vi "Day_File_Plotter.vi"() -> ()   [LabVIEW 2012]
uses:
  Anemometry/Anemometry Sub Vis/File/Setup_Filetype.ctl
panel:
  in  "Reload":bool
  out "Setup exists?":bool
  out "Plot 3 status":string
  out "Plot 2 status":string
  out "Plot 1 status":string
  out "Change Scale?":bool
  out "Min Memory":timestamp
  out "Max Memory":timestamp
  in  "Show Full Time?":bool
  in  "Max Time":timestamp format="%<%H:%M\n%x>T"
  in  "Min Time":timestamp format="%<%H:%M\n%x>T"
  out "Plot 3 Chs":string[](array[string])
  out "Plot 2 Chs":string[](array[string])
  out "Plot 1 Chs":string[](array[string])
  in  "Save plot number":T1(ring)
  in  "Data folder location":path
  in  "Save 3":bool
  in  "Save 2":bool
  in  "Save 1":bool
  in  "Averaging Time (min)":dbl=1.0 min=0.0 format="%#.2f"
  in  "End Date":timestamp format="%<%x>T"
  in  "Selector 1":i32[](listbox)
  in  "Search 1":string
  in  "Search 2":string
  in  "Search 3":string
  out "Last Updated":string
  out "Plot 3":cluster{"Times":dbl[], "Output array":dbl[]}[](graph)
  in  "Selector 3":i32[](listbox)
  out "Plot 2":cluster{"Times":dbl[], "Output array":dbl[]}[](graph)
  in  "Selector 2":i32[](listbox)
  in  "stop":bool
  out "Plot 1":cluster{dbl[], "Output array":dbl[]}[](graph)
  in  "History (days)":i32 min=0
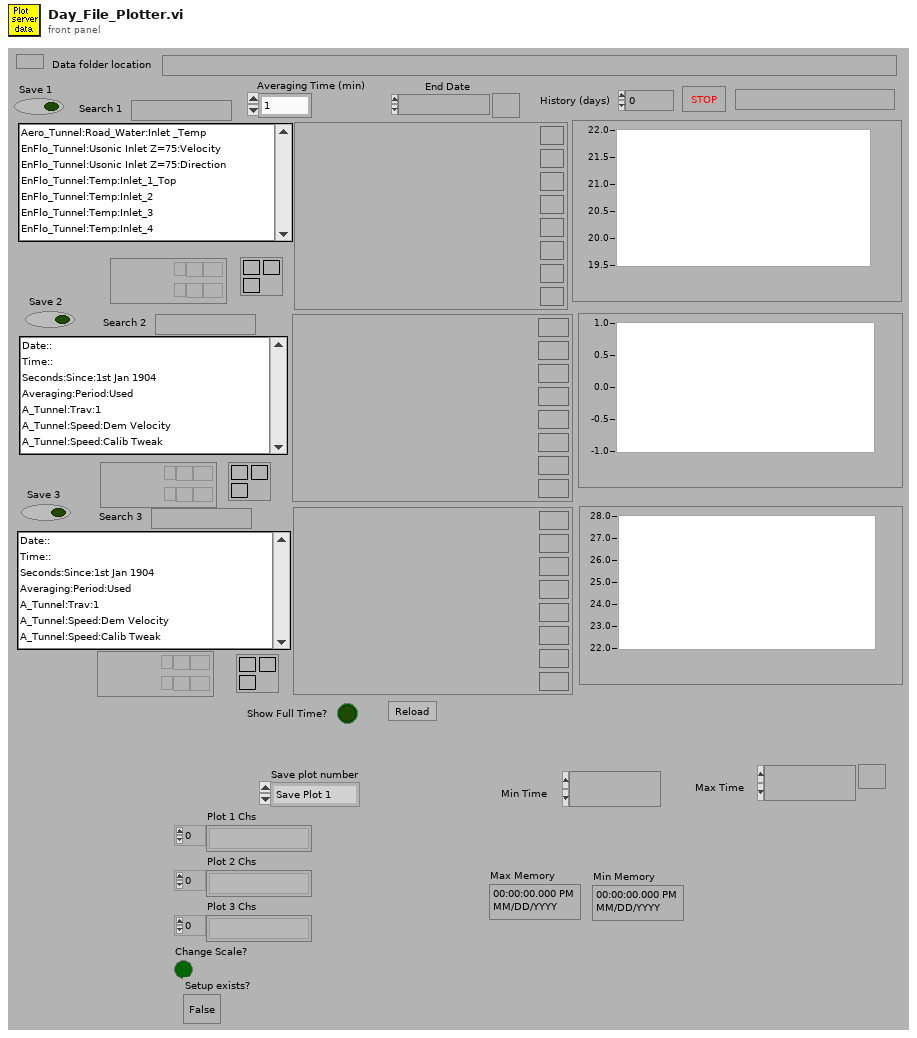
[diagram p1: front panel]
types:
  T1 = enum16{"Save Plot 1", "Save Plot 2", "Save Plot 3"}
  T2 = typedef "Setup_Filetype.ctl" = enum16{"Measurement Setups", "Calibration Setups", "General", "Results File Plotter Setups", "Speed Calib Tweaks"}
  T3 = enum32{"existing file", "new file", "new or existing file", "existing dir", "new dir", "new or existing dir", "existing file (use LLBs)", "new file (use LLBs)", "new or existing file (use LLBs)", "new or existing file or directory (use LLBs)"}
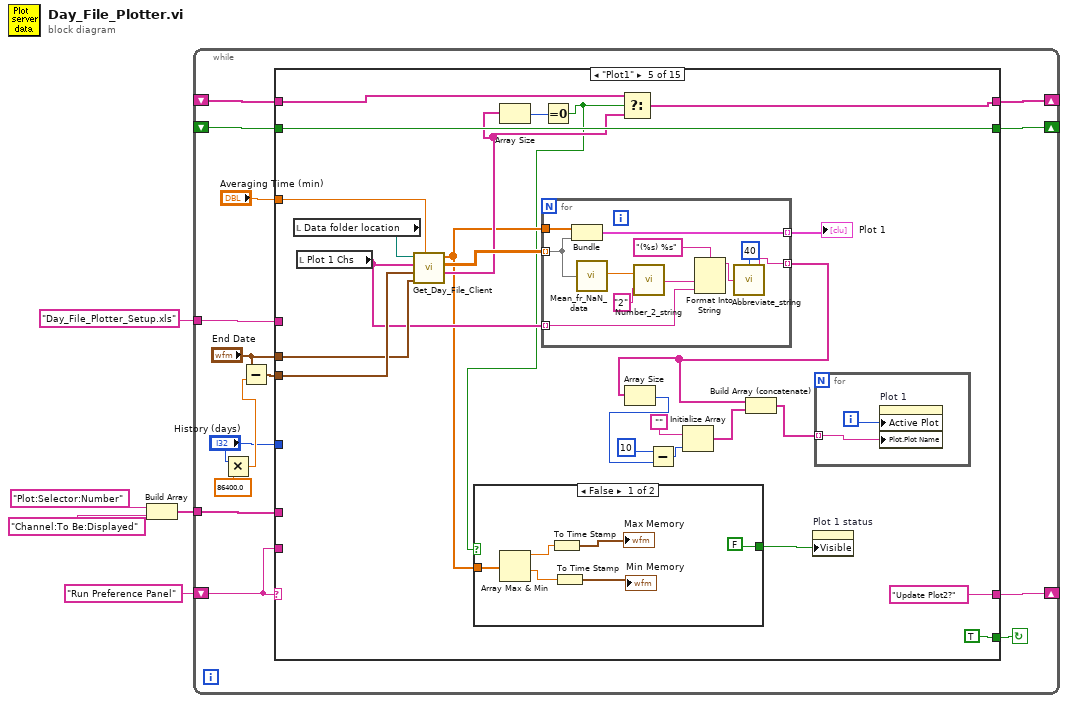
[diagram p0: block diagram]
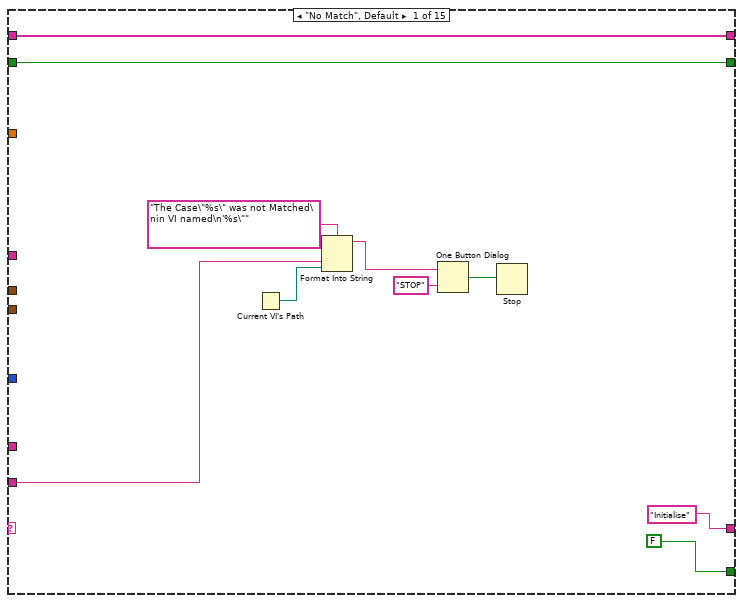
[diagram p2: hidden frame]
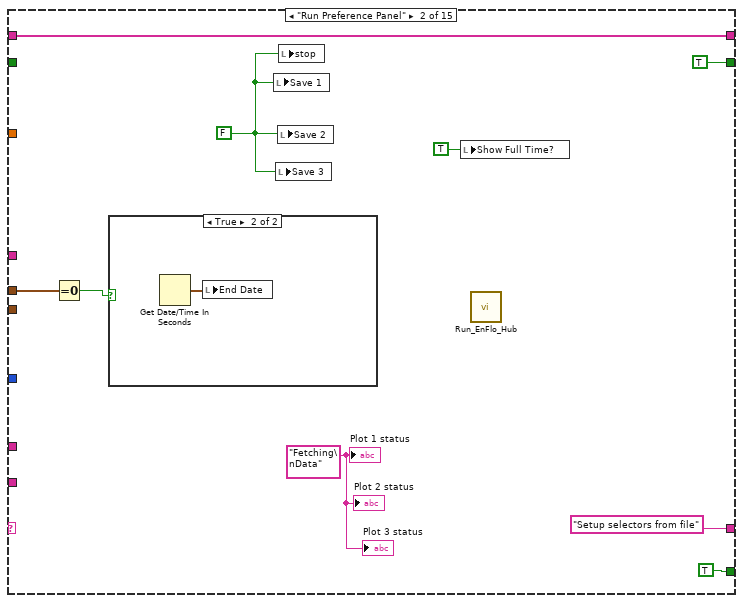
[diagram p3: hidden frame]
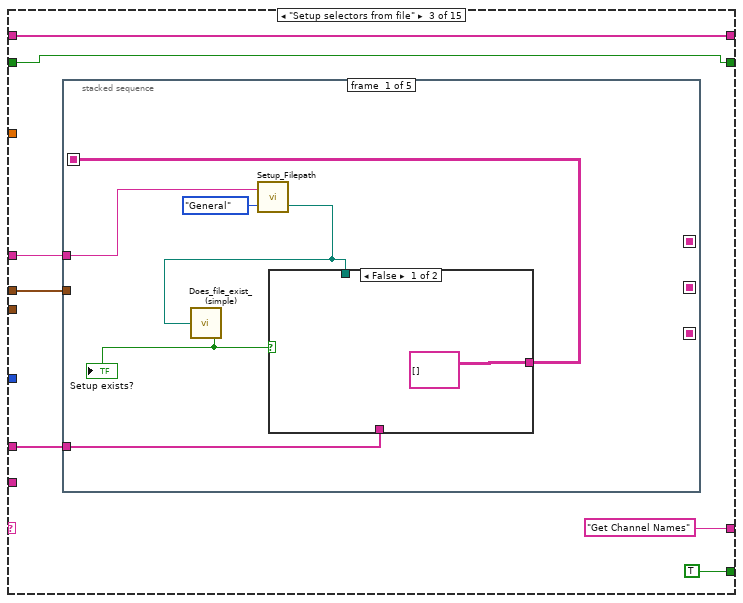
[diagram p5: hidden frame]
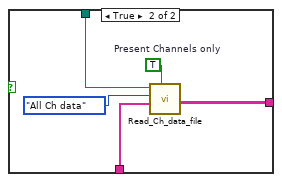
[diagram p6: hidden frame]
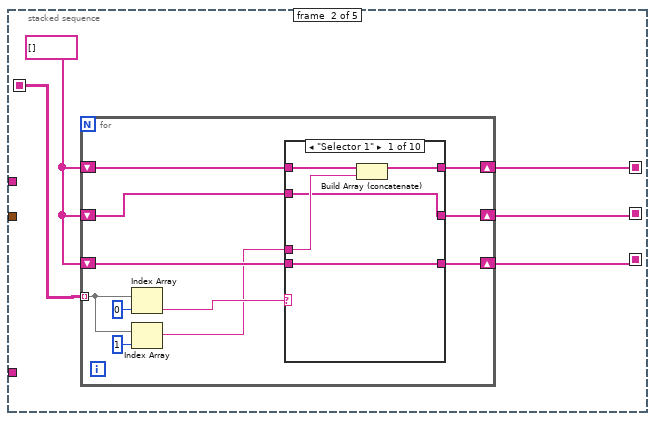
[diagram p7: hidden frame]
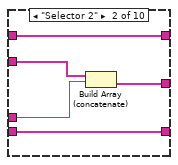
[diagram p8: hidden frame]
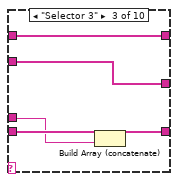
[diagram p9: hidden frame]
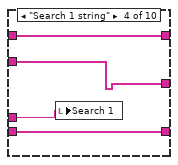
[diagram p10: hidden frame]
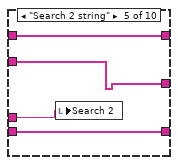
[diagram p11: hidden frame]
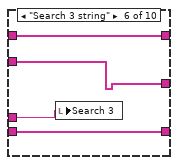
[diagram p12: hidden frame]
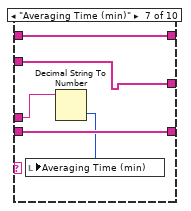
[diagram p13: hidden frame]
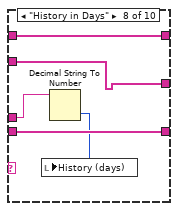
[diagram p14: hidden frame]
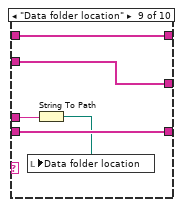
[diagram p15: hidden frame]
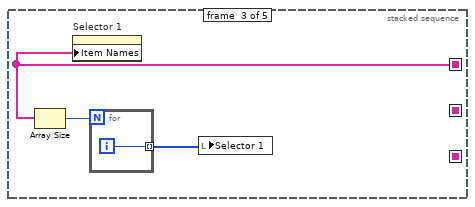
[diagram p17: hidden frame]
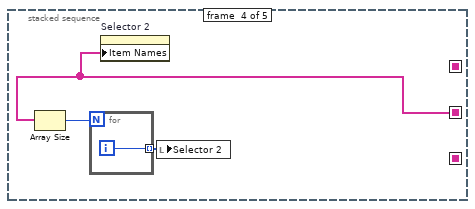
[diagram p18: hidden frame]
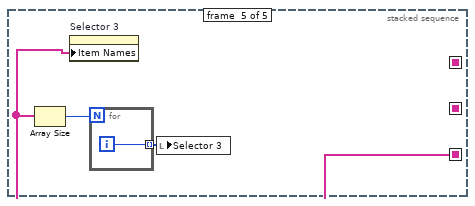
[diagram p19: hidden frame]
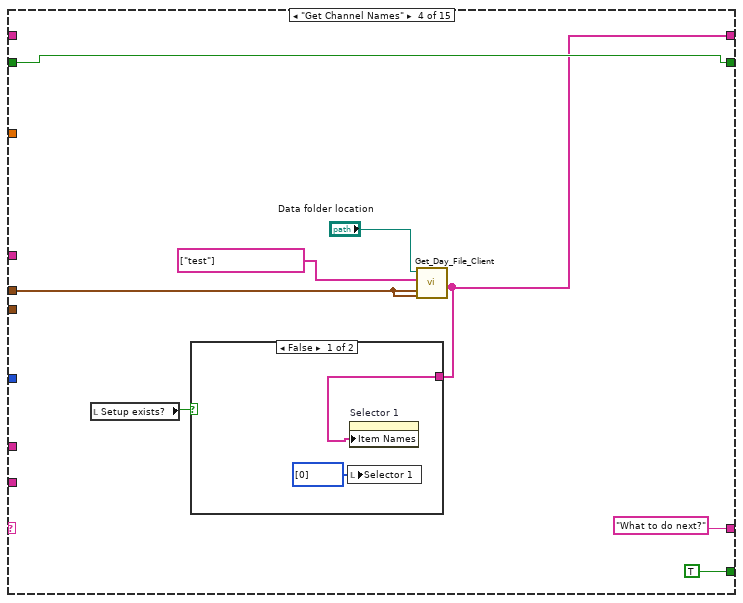
[diagram p20: hidden frame]
diagram:
  n1 = Build Array("Plot:Selector:Number", "Channel:To Be:Displayed") -> (w2:string[])
  n2 = while {
    shift-left: "Run Preference Panel" -> [w18]
    shift-right: [w19] -> _
    tunnel: w2 -> [w17]
    tunnel: "Day_File_Plotter_Setup.xls" -> [w16]
    shift-right: [w11] -> _
    shift-left: _ -> [w10]
    shift-right: [w7] -> _
    shift-left: _ -> [w6]
    stop <- w20 continue-if-true
    n3 = Multiply(x="History (days)", y=86400.0) -> (x*y=w14:dbl)
    n4 = Subtract(x="End Date", y=w14) -> (x-y=w13:timestamp)
    n5 = case shown="\"Plot1\"" w18 {
      tunnel: [FALSE TRUE TRUE TRUE TRUE TRUE TRUE TRUE TRUE TRUE TRUE TRUE TRUE TRUE w607] -> w20
      tunnel: ["Initialise" "Setup selectors from file" "Get Channel Names" "What to do next?" "Update Plot2?" "Update Plot3?" "Rescale plots?" "Update Plot1?" w314 w366 w420 w472 w568 w591 "Check for Zoom" ("t")] -> w19
      tunnel: w18 -> [w25 _ _ _ _ _ _ _ _ _ _ _ _ _ _]
      tunnel: w17 -> [_ _ w44 _ _ _ _ _ _ _ _ _ _ _ w614]
      tunnel: w16 -> [_ _ w45 _ _ _ _ _ _ _ _ _ _ _ w613]
      tunnel: w13 -> [_ _ _ _ w161 w206 w251 _ _ _ _ _ _ _ _]
      tunnel: "End Date" -> [_ w36 w42 w137 w160 w205 w250 _ _ _ _ _ w561 _ _]
      tunnel: [w22 TRUE w43 w138 w164 w209 w254 w282 w331 w384 w437 w473 w560 w590 w611] -> w11
      tunnel: w10 -> [w22 _ w43 w138 w164 w209 w254 w282 w331 w384 w437 w473 _ w589 w611]
      tunnel: "History (days)" -> [_ _ _ _ _ _ _ _ _ _ _ _ _ _ w605]
      tunnel: "Averaging Time (min)" -> [_ _ _ _ w163 w208 w253 _ _ _ _ _ w559 _ w610]
      tunnel: [w21 w34 w41 w134 w155 w200 w245 w283 w327 w380 w433 w474 w557 w596 w609] -> w7
      tunnel: w6 -> [w21 w34 w41 _ w157 w202 w247 w283 w327 w380 w433 w474 w557 w596 w609]
      frame "No Match", Default {
        n6 = Current VI's Path() -> (path=w24:path)
        n7 = Format Into String(format string="The Case\"%s\" was not Matched\nin VI named\n'%s\"" ("Format String"), w25, w24) -> (resulting string=w28:string)  [unwired: 2 in, 1 out]
        n8 = One Button Dialog(message=w28, button name ("OK")="STOP") -> (true=w26:bool)
        n9 = Stop(stop? (T)=w26) -> ()
      }
      frame "Run Preference Panel" {
        w31 = "Fetching\nData" ("Plot 1 status")
        w33 = FALSE
        n10 = Equal To 0?(x=w36) -> (x = 0?=w35:bool)
        n11 = case shown="True" w35 {
          frame False {
          }
          frame True {
            n12 = Get Date/Time In Seconds() -> (seconds since 1Jan1904=w40:timestamp)
            n13 = local write "End Date"(w40) -> ()
          }
        }
        n14 = local write "Save 1"(w33) -> ()
        n15 = local write "Save 3"(w33) -> ()
        n16 = local write "Save 2"(w33) -> ()
        n17 = local write "stop"(w33) -> ()
        n18 = local write "Show Full Time?"(TRUE ("Show Full Time?")) -> ()
        n19 = call "Run_EnFlo_Hub.vi"() -> ()  [unwired: 8 out]
        "Plot 1 status" <- w31
        "Plot 3 status" <- w31
        "Plot 2 status" <- w31
      }
      frame "Setup selectors from file" {
        n20 = stacked-sequence {
          seq-local: [w52 _ _ _ _] -> [_ w64 _ _ _]
          seq-local: [_ w62 _ _ _] -> [_ _ w123 _ _]
          seq-local: [_ w60 _ _ _] -> [_ _ _ w125 _]
          seq-local: [_ w61 _ _ _] -> [_ _ _ _ w129]
          tunnel: w45 -> [w49 _ _ _ _]
          tunnel: w44 -> [w53 _ _ _ _]
          tunnel: w42 -> [_ _ _ _ _]
          frame #0 {
            n21 = call "Setup_Filepath.vi"("Setup File Type"=Setup_Filetype."General", "Filename in"=w49) -> ("Filename Out"=w48:path)  [unwired: 1 out]
            n22 = call "Does_file_exist_(simple).vi"("Pathname"=w48) -> ("exists?"=w51:bool)
            "Setup exists?" <- w51
            n23 = case shown="False" w51 {
              tunnel: w48 -> [_ w59]
              tunnel: w53 -> [_ w58]
              tunnel: [string[][] [] ("Channel Values") w55] -> w52
              frame False {
              }
              frame True {
                w57 = TRUE  # Present Channels only
                n24 = call "Read_Ch_data_file.vi"("Present Channels only"=w57, "Present Channels"=w58, "Output"=enum16{"All Ch data", "The last few rows"}."All Ch data", "Filename"=w59) -> ("Channel Values"=w55:string[][])  [unwired: 1 in, 4 out]
              }
            }
          }
          frame #1 {
            w63 = string[] []
            n25 = for {
              shift-right: [w70] -> w62
              shift-left: w63 -> [w71]
              tunnel: w64 -> [w72] mode=indexing
              shift-right: [w68] -> w60
              shift-left: w63 -> [w69]
              shift-right: [w66] -> w61
              shift-left: w63 -> [w67]
              n26 = Index Array(array=w72, index=0 ("Index")) -> (element=w74:string)
              n27 = Index Array(array=w72, index=1 ("Index")) -> (element=w65:string)
              n28 = case shown="\"Selector 1\"" w74 {
                tunnel: w71 -> [w80 w85 w86 w94 w98 w102 w107 w108 w115 w120]
                tunnel: [w79 w85 w86 w94 w98 w102 w107 w108 w115 w120] -> w70
                tunnel: w65 -> [w78 w82 w88 w91 w95 w99 w104 w110 w114 _]
                tunnel: w69 -> [w77 w83 w87 w93 w97 w101 w106 w112 w117 w119]
                tunnel: [w77 w81 w87 w93 w97 w101 w106 w112 w117 w119] -> w68
                tunnel: w67 -> [w76 w84 w90 w92 w96 w100 w105 w111 w116 w118]
                tunnel: [w76 w84 w89 w92 w96 w100 w105 w111 w116 w118] -> w66
                frame "Selector 1" {
                  n29 = Build Array (concatenate)(w80, w78) -> (w79:string[])
                }
                frame "Selector 2" {
                  n30 = Build Array (concatenate)(w83, w82) -> (w81:string[])
                }
                frame "Selector 3" {
                  n31 = Build Array (concatenate)(w90, w88) -> (w89:string[])
                }
                frame "Search 1 string" {
                  n32 = local write "Search 1"(w91) -> ()
                }
                frame "Search 2 string" {
                  n33 = local write "Search 2"(w95) -> ()
                }
                frame "Search 3 string" {
                  n34 = local write "Search 3"(w99) -> ()
                }
                frame "Averaging Time (min)" {
                  n35 = Decimal String To Number(string=w104) -> (number=w103:i32)  [unwired: 3 out]
                  n36 = local write "Averaging Time (min)"(w103) -> ()
                }
                frame "History in Days" {
                  n37 = Decimal String To Number(string=w110) -> (number=w109:i32)  [unwired: 3 out]
                  n38 = local write "History (days)"(w109) -> ()
                }
                frame "Data folder location" {
                  n39 = String To Path(string=w114) -> (path=w113:path)
                  n40 = local write "Data folder location"(w113) -> ()
                }
                frame "No match", Default {
                }
              }
            }
          }
          frame #2 {
            n41 = Array Size(array=w123) -> (size(s)=w122:i32)
            n42 = property on="Selector 1" class="LstBox (strict)"("Item Names"=w123) -> ()  [unwired: 2 in, 2 out]
            n43 = for {
              N: w122 -> [_]
              tunnel: [w124] -> w121 mode=indexing
              i -> [w124]
            }
            n44 = local write "Selector 1"(w121) -> ()
          }
          frame #3 {
            n45 = Array Size(array=w125) -> (size(s)=w127:i32)
            n46 = for {
              N: w127 -> [_]
              tunnel: [w128] -> w126 mode=indexing
              i -> [w128]
            }
            n47 = property on="Selector 2" class="LstBox (strict)"("Item Names"=w125) -> ()  [unwired: 2 in, 2 out]
            n48 = local write "Selector 2"(w126) -> ()
          }
          frame #4 {
            n49 = Array Size(array=w129) -> (size(s)=w131:i32)
            n50 = property on="Selector 3" class="LstBox (strict)"("Item Names"=w129) -> ()  [unwired: 2 in, 2 out]
            n51 = for {
              N: w131 -> [_]
              tunnel: [w132] -> w130 mode=indexing
              i -> [w132]
            }
            n52 = local write "Selector 3"(w130) -> ()
          }
        }
      }
      frame "Get Channel Names" {
        n53 = local read "Setup exists?"() -> (w133:bool)
        n54 = call "Get_Day_File_Client.vi"("End time"=w137, "Start time"=w137, "Channel Names"=string[] ["test"], "Data folder location"="Data folder location") -> ("All Channel Names"=w134:string[])  [unwired: 1 in, 3 out]
        n55 = case shown="False" w133 {
          tunnel: w134 -> [w142 _]
          frame False {
            n56 = local write "Selector 1"(i32[] [0] ("Selector 1")) -> ()
            n57 = property on="Selector 1" class="LstBox (strict)"("Item Names"=w142) -> ()  [unwired: 2 in, 2 out]
          }
          frame True {
          }
        }
      }
      frame "Plot1" {
        n58 = local read "Data folder location"() -> (w162:path)
        n59 = local read "Plot 1 Chs"() -> (w147:string[])
        n60 = call "Get_Day_File_Client.vi"("Averaging Time (min)"=w163, "End time"=w160, "Start time"=w161, "Channel Names"=w147, "Data folder location"=w162) -> ("All Channel Names"=w156:string[], "Data"=w159:dbl[][], "Times"=w145:dbl[])  [unwired: 1 out]
        n61 = Array Size(array=w156) -> (size(s)=w158:i32)
        n62 = for {
          tunnel: w159 -> [w175] mode=indexing
          tunnel: [w184] -> w154 mode=indexing
          tunnel: w145 -> [w183]
          tunnel: [w179] -> w146 mode=indexing
          tunnel: w147 -> [w176] mode=indexing
          n63 = Bundle("Times"=w183, "Data"=w175) -> (w184:cluster{"Times":dbl[], "Data":dbl[]})  [unwired: 1 out]
          n64 = call "Mean_fr_NaN_data.vi"("Data"=w175) -> ("Mean value"=w174:dbl)  [unwired: 1 out]
          n65 = call "Number_2_string.vi"("precision"="2", "number"=w174) -> ("String"=w177:string)
          n66 = Format Into String(format string="(%s) %s", w177, w176) -> (resulting string=w180:string)  [unwired: 2 in, 1 out]
          n67 = call "Abbreviate_string.vi"("Input String"=w180, "Max String Length"=40) -> ("Output String"=w179:string)
        }
        "Plot 1" <- w154
        n68 = Equal To 0?(x=w158) -> (x = 0?=w144:bool)
        n69 = case shown="False" w144 {
          tunnel: w145 -> [w172 _]
          tunnel: [FALSE ("Visible") FALSE ("Visible")] -> w143
          frame False {
            n70 = Array Max & Min(array=w172) -> (max value=w171:dbl, min value=w169:dbl)  [unwired: 2 out]
            n71 = To Time Stamp(1:w171) -> (0:→"Max Memory":timestamp)
            n72 = To Time Stamp(1:w169) -> (0:→"Min Memory":timestamp)
          }
          frame True {
          }
        }
        n73 = Select(t=w157, s=w144, f=w156) -> (s? t:f=w155:string[])
        n74 = Array Size(array=w146) -> (size(s)=w152:i32)
        n75 = Subtract(x=10 ("dimension size"), y=w152) -> (x-y=w153:i32)
        n76 = Initialize Array("", w153) -> (w150:string[])
        n77 = Build Array (concatenate)(w146, w150) -> (w148:string[])
        n78 = property on="Plot 1 status" class="Str"("Visible"=w143) -> ()  [unwired: 2 in, 2 out]
        n79 = for {
          tunnel: w148 -> [w185] mode=indexing
          i -> [w186]
          n80 = property on="Plot 1" class="XYGraph (strict)"("Active Plot"=w186, "Plot.Plot Name"=w185) -> ()  [unwired: 2 in, 2 out]
        }
      }
      frame "Plot2" {
        n81 = local read "Plot 2 Chs"() -> (w193:string[])
        n82 = local read "Data folder location"() -> (w207:path)
        n83 = call "Get_Day_File_Client.vi"("Averaging Time (min)"=w208, "End time"=w205, "Start time"=w206, "Channel Names"=w193, "Data folder location"=w207) -> ("All Channel Names"=w201:string[], "Data"=w204:dbl[][], "Times"=w190:dbl[])  [unwired: 1 out]
        n84 = Array Size(array=w201) -> (size(s)=w203:i32)
        n85 = for {
          tunnel: w204 -> [w220] mode=indexing
          tunnel: [w229] -> w192 mode=indexing
          tunnel: w190 -> [w228]
          tunnel: [w224] -> w191 mode=indexing
          tunnel: w193 -> [w221] mode=indexing
          n86 = Bundle("Times"=w228, "Data"=w220) -> (w229:cluster{"Times":dbl[], "Data":dbl[]})  [unwired: 1 out]
          n87 = call "Mean_fr_NaN_data.vi"("Data"=w220) -> ("Mean value"=w219:dbl)  [unwired: 1 out]
          n88 = call "Number_2_string.vi"("precision"="2", "number"=w219) -> ("String"=w222:string)
          n89 = Format Into String(format string="(%s) %s", w222, w221) -> (resulting string=w225:string)  [unwired: 2 in, 1 out]
          n90 = call "Abbreviate_string.vi"("Input String"=w225, "Max String Length"=40) -> ("Output String"=w224:string)
        }
        "Plot 2" <- w192
        n91 = Equal To 0?(x=w203) -> (x = 0?=w189:bool)
        n92 = case shown="True" w189 {
          tunnel: w190 -> [w213 _]
          tunnel: [w212 w218] -> w188
          tunnel: FALSE -> [w212 w218]
          frame False {
            n93 = Array Max & Min(array=w213) -> (max value=w217:dbl, min value=w216:dbl)  [unwired: 2 out]
            n94 = To Time Stamp(1:w217) -> (0:w214:timestamp)
            n95 = To Time Stamp(1:w216) -> (0:w215:timestamp)
            n96 = local write "Max Memory"(w214) -> ()
            n97 = local write "Min Memory"(w215) -> ()
          }
          frame True {
          }
        }
        n98 = Array Size(array=w191) -> (size(s)=w198:i32)
        n99 = Select(t=w202, s=w189, f=w201) -> (s? t:f=w200:string[])
        n100 = Subtract(x=10 ("dimension size"), y=w198) -> (x-y=w199:i32)
        n101 = Initialize Array("", w199) -> (w196:string[])
        n102 = Build Array (concatenate)(w191, w196) -> (w194:string[])
        n103 = property on="Plot 2 status" class="Str"("Visible"=w188) -> ()  [unwired: 2 in, 2 out]
        n104 = for {
          tunnel: w194 -> [w230] mode=indexing
          i -> [w231]
          n105 = property on="Plot 2" class="XYGraph (strict)"("Active Plot"=w231, "Plot.Plot Name"=w230) -> ()  [unwired: 2 in, 2 out]
        }
      }
      frame "Plot3" {
        n106 = local read "Plot 3 Chs"() -> (w238:string[])
        n107 = local read "Data folder location"() -> (w252:path)
        n108 = call "Get_Day_File_Client.vi"("Averaging Time (min)"=w253, "End time"=w250, "Start time"=w251, "Channel Names"=w238, "Data folder location"=w252) -> ("All Channel Names"=w246:string[], "Data"=w249:dbl[][], "Times"=w235:dbl[])  [unwired: 1 out]
        n109 = Array Size(array=w246) -> (size(s)=w248:i32)
        n110 = for {
          tunnel: w249 -> [w265] mode=indexing
          tunnel: [w274] -> w237 mode=indexing
          tunnel: w235 -> [w273]
          tunnel: [w269] -> w236 mode=indexing
          tunnel: w238 -> [w266] mode=indexing
          n111 = Bundle("Times"=w273, "Data"=w265) -> (w274:cluster{"Times":dbl[], "Data":dbl[]})  [unwired: 1 out]
          n112 = call "Mean_fr_NaN_data.vi"("Data"=w265) -> ("Mean value"=w264:dbl)  [unwired: 1 out]
          n113 = call "Number_2_string.vi"("precision"="2", "number"=w264) -> ("String"=w267:string)
          n114 = Format Into String(format string="(%s) %s", w267, w266) -> (resulting string=w270:string)  [unwired: 2 in, 1 out]
          n115 = call "Abbreviate_string.vi"("Input String"=w270, "Max String Length"=40) -> ("Output String"=w269:string)
        }
        "Plot 3" <- w237
        n116 = Equal To 0?(x=w248) -> (x = 0?=w234:bool)
        n117 = case shown="True" w234 {
          tunnel: w235 -> [w258 _]
          tunnel: [w257 w263] -> w233
          tunnel: FALSE -> [w257 w263]
          frame False {
            n118 = Array Max & Min(array=w258) -> (max value=w262:dbl, min value=w261:dbl)  [unwired: 2 out]
            n119 = To Time Stamp(1:w262) -> (0:w259:timestamp)
            n120 = To Time Stamp(1:w261) -> (0:w260:timestamp)
            n121 = local write "Max Memory"(w259) -> ()
            n122 = local write "Min Memory"(w260) -> ()
          }
          frame True {
          }
        }
        n123 = Array Size(array=w236) -> (size(s)=w243:i32)
        n124 = Select(t=w247, s=w234, f=w246) -> (s? t:f=w245:string[])
        n125 = Subtract(x=10 ("dimension size"), y=w243) -> (x-y=w244:i32)
        n126 = Initialize Array("", w244) -> (w241:string[])
        n127 = Build Array (concatenate)(w236, w241) -> (w239:string[])
        n128 = property on="Plot 3 status" class="Str"("Visible"=w233) -> ()  [unwired: 2 in, 2 out]
        n129 = for {
          tunnel: w239 -> [w275] mode=indexing
          i -> [w276]
          n130 = property on="Plot 3" class="XYGraph (strict)"("Active Plot"=w276, "Plot.Plot Name"=w275) -> ()  [unwired: 2 in, 2 out]
        }
      }
      frame "Check for Zoom" {
        n131 = local read "Change Scale?"() -> (w278:bool)
        n132 = Or(x=w278, y="Show Full Time?") -> (x .or. y?=w277:bool)
        n133 = case shown="False" w277 {
          frame False {
            n134 = local read "Max Time"() -> (w290:timestamp)
            n135 = local read "Min Time"() -> (w291:timestamp)
            n136 = To Double Precision Float(number=w290) -> (double precision float=w289:dbl)
            n137 = To Double Precision Float(number=w291) -> (double precision float=w288:dbl)
            n138 = while {
              tunnel: w289 -> [w300]
              tunnel: w288 -> [w299]
              tunnel: [w293] -> w287
              tunnel: [w292] -> w286
              i -> [w302]
              stop <- w294 continue-if-true
              n139 = Increment(x=w302) -> (x+1=w301:i32)
              n140 = case shown="3" w301 {
                tunnel: [w305 w307 w310] -> w293
                tunnel: [w304 w306 w309] -> w292
                tunnel: [TRUE TRUE FALSE] -> w295
                frame 1, Default {
                  n141 = property on="Plot 1" class="XYGraph (strict)"() -> ("X Scale.Range:Maximum"=w305:dbl, "X Scale.Range:Minimum"=w304:dbl)  [unwired: 2 in, 2 out]
                }
                frame 2 {
                  n142 = property on="Plot 2" class="XYGraph (strict)"() -> ("X Scale.Range:Maximum"=w307:dbl, "X Scale.Range:Minimum"=w306:dbl)  [unwired: 2 in, 2 out]
                }
                frame 3 {
                  n143 = property on="Plot 3" class="XYGraph (strict)"() -> ("X Scale.Range:Maximum"=w310:dbl, "X Scale.Range:Minimum"=w309:dbl)  [unwired: 2 in, 2 out]
                }
              }
              n144 = Equal?(x=w300, y=w293) -> (x = y?=w297:bool)
              n145 = Equal?(x=w292, y=w299) -> (x = y?=w298:bool)
              n146 = And(x=w297, y=w298) -> (x .and. y?=w296:bool)
              n147 = And(x=w296, y=w295) -> (x .and. y?=w294:bool)
            }
            n148 = To Time Stamp(1:w287) -> (0:w284:timestamp)
            n149 = To Time Stamp(1:w286) -> (0:w285:timestamp)
            n150 = local write "Max Time"(w284) -> ()
            n151 = local write "Min Time"(w285) -> ()
          }
          frame True {
          }
        }
      }
      frame "Update Plot1?" {
        n152 = property on="Selector 1" class="LstBox (strict)"() -> ("Item Names"=w325:string[])  [unwired: 2 in, 2 out]
        n153 = case shown="True" "Save 1" {
          tunnel: ["Update Plot2?" "Save Plot" ("t")] -> w312
          frame False {
          }
          frame True {
            n154 = local write "Save plot number"(T1."Save Plot 1" ("Save plot number")) -> ()
          }
        }
        n155 = for {
          tunnel: w327 -> [w354]
          shift-right: [w349] -> w326
          shift-left: string[] [] -> [w350]
          tunnel: w325 -> [w352]
          tunnel: "Selector 1" -> [w351] mode=indexing
          n156 = Index Array(array=w352, index=w351) -> (element=w348:string)
          n157 = Search 1D Array(1D array=w354, element=w348) -> (index of element=w353:i32)  [unwired: 1 out]
          n158 = case shown="0, Default" w353 {
            tunnel: w353 -> [_ _]
            tunnel: w350 -> [w357 w358]
            tunnel: [w356 w358] -> w349
            tunnel: w348 -> [w355 _]
            frame 0, Default {
              n159 = Build Array (concatenate)(w357, w355) -> (w356:string[])
            }
            frame -1 {
            }
          }
        }
        "Plot 1 Chs" <- w326
        n160 = while {
          shift-right: [w359] -> w334
          shift-left: _ -> [w364]
          tunnel: [w364] -> w333
          shift-right: [w361] -> _
          shift-left: _ -> [w362]
          tunnel: w331 -> [w361]
          tunnel: [w360] -> w330
          tunnel: w326 -> [w359]
          stop <- FALSE continue-if-true
          n161 = Not Equal?(x=w362, y=w361) -> (x != y?=w360:bool)
        }
        n162 = Not Equal?(x=w333, y=w334) -> (x != y?=w332:bool)
        n163 = And(x=w331, y=w330) -> (x .and. y?=w329:bool)
        n164 = Compound Arithmetic op=OR(w329, w332) -> (w313:bool)
        n165 = case shown="True" w313 {
          tunnel: [w336 "Plot1"] -> w314
          tunnel: w312 -> [w336 _]
          frame False {
          }
          frame True {
            n166 = property on="Plot 1 status" class="Str"("Visible"=TRUE) -> ()  [unwired: 2 in, 2 out]
          }
        }
        n167 = call "Selection_with_Search.vi"("Selected Channel Names"=w326, "Search String"="Search 1", "All Channel Names"=w327) -> ("Item Names"=w322:string[])
        n168 = for {
          tunnel: w322 -> [w347]
          tunnel: w326 -> [w346] mode=indexing
          tunnel: [w345] -> w323 mode=indexing
          n169 = Search 1D Array(1D array=w347, element=w346) -> (index of element=w345:i32)  [unwired: 1 out]
        }
        n170 = Not Equal?(x=w322, y=w325) -> (x != y?=w324:bool)
        n171 = To Double Precision Float(number="Max Time") -> (double precision float=w317:dbl)
        n172 = To Double Precision Float(number="Min Time") -> (double precision float=w315:dbl)
        n173 = case shown="True" w324 {
          tunnel: w323 -> [_ w344]
          tunnel: w322 -> [_ w343]
          frame False {
          }
          frame True {
            n174 = local write "Selector 1"(w344) -> ()
            n175 = property on="Selector 1" class="LstBox (strict)"("Item Names"=w343, "Top Row"=0) -> ()  [unwired: 2 in, 2 out]
          }
        }
        n176 = property on="Plot 1" class="XYGraph (strict)"("X Scale.Range:Maximum"=w317, "X Scale.Range:Minimum"=w315) -> ()  [unwired: 2 in, 2 out]
      }
      frame "Update Plot2?" {
        n177 = property on="Selector 2" class="LstBox (strict)"() -> ("Item Names"=w375:string[])  [unwired: 2 in, 2 out]
        n178 = case shown="True" "Save 2" {
          tunnel: ["Update Plot3?" "Save Plot" ("t")] -> w365
          frame False {
          }
          frame True {
            n179 = local write "Save plot number"(T1."Save Plot 2" ("Save plot number")) -> ()
          }
        }
        n180 = for {
          tunnel: w380 -> [w407]
          shift-right: [w402] -> w379
          shift-left: string[] [] -> [w403]
          tunnel: w375 -> [w405]
          tunnel: "Selector 2" -> [w404] mode=indexing
          n181 = Index Array(array=w405, index=w404) -> (element=w401:string)
          n182 = Search 1D Array(1D array=w407, element=w401) -> (index of element=w406:i32)  [unwired: 1 out]
          n183 = case shown="0, Default" w406 {
            tunnel: w406 -> [_ _]
            tunnel: w403 -> [w410 w411]
            tunnel: [w409 w411] -> w402
            tunnel: w401 -> [w408 _]
            frame 0, Default {
              n184 = Build Array (concatenate)(w410, w408) -> (w409:string[])
            }
            frame -1 {
            }
          }
        }
        "Plot 2 Chs" <- w379
        n185 = while {
          shift-right: [w412] -> w387
          shift-left: _ -> [w417]
          tunnel: [w417] -> w386
          shift-right: [w414] -> _
          shift-left: _ -> [w415]
          tunnel: w384 -> [w414]
          tunnel: [w413] -> w383
          tunnel: w379 -> [w412]
          stop <- FALSE continue-if-true
          n186 = Not Equal?(x=w415, y=w414) -> (x != y?=w413:bool)
        }
        n187 = Not Equal?(x=w386, y=w387) -> (x != y?=w385:bool)
        n188 = And(x=w384, y=w383) -> (x .and. y?=w382:bool)
        n189 = local read "Max Time"() -> (w370:timestamp)
        n190 = local read "Min Time"() -> (w371:timestamp)
        n191 = Compound Arithmetic op=OR(w382, w385) -> (w367:bool)
        n192 = To Double Precision Float(number=w370) -> (double precision float=w369:dbl)
        n193 = To Double Precision Float(number=w371) -> (double precision float=w368:dbl)
        n194 = case shown="True" w367 {
          tunnel: [w389 "Plot2"] -> w366
          tunnel: w365 -> [w389 _]
          frame False {
          }
          frame True {
            n195 = property on="Plot 2 status" class="Str"("Visible"=TRUE) -> ()  [unwired: 2 in, 2 out]
          }
        }
        n196 = call "Selection_with_Search.vi"("Selected Channel Names"=w379, "Search String"="Search 2", "All Channel Names"=w380) -> ("Item Names"=w376:string[])
        n197 = for {
          tunnel: w376 -> [w400]
          tunnel: w379 -> [w399] mode=indexing
          tunnel: [w398] -> w377 mode=indexing
          n198 = Search 1D Array(1D array=w400, element=w399) -> (index of element=w398:i32)  [unwired: 1 out]
        }
        n199 = property on="Plot 2" class="XYGraph (strict)"("X Scale.Range:Maximum"=w369, "X Scale.Range:Minimum"=w368) -> ()  [unwired: 2 in, 2 out]
        n200 = Not Equal?(x=w376, y=w375) -> (x != y?=w378:bool)
        n201 = case shown="True" w378 {
          tunnel: w377 -> [_ w397]
          tunnel: w376 -> [_ w396]
          frame False {
          }
          frame True {
            n202 = property on="Selector 2" class="LstBox (strict)"("Item Names"=w396, "Top Row"=0) -> ()  [unwired: 2 in, 2 out]
            n203 = local write "Selector 2"(w397) -> ()
          }
        }
      }
      frame "Update Plot3?" {
        n204 = property on="Selector 3" class="LstBox (strict)"() -> ("Item Names"=w425:string[])  [unwired: 2 in, 2 out]
        n205 = case shown="False" "Save 3" {
          tunnel: ["Rescale plots?" "Save Plot" ("t")] -> w418
          frame False {
          }
          frame True {
            n206 = local write "Save plot number"(T1."Save Plot 3" ("Save plot number")) -> ()
          }
        }
        n207 = for {
          tunnel: w433 -> [w460]
          shift-right: [w455] -> w432
          shift-left: string[] [] -> [w456]
          tunnel: w425 -> [w458]
          tunnel: "Selector 3" -> [w457] mode=indexing
          n208 = Index Array(array=w458, index=w457) -> (element=w454:string)
          n209 = Search 1D Array(1D array=w460, element=w454) -> (index of element=w459:i32)  [unwired: 1 out]
          n210 = case shown="0, Default" w459 {
            tunnel: w459 -> [_ _]
            tunnel: w456 -> [w463 w464]
            tunnel: [w462 w464] -> w455
            tunnel: w454 -> [w461 _]
            frame 0, Default {
              n211 = Build Array (concatenate)(w463, w461) -> (w462:string[])
            }
            frame -1 {
            }
          }
        }
        "Plot 3 Chs" <- w432
        n212 = while {
          shift-right: [w465] -> w440
          shift-left: _ -> [w470]
          tunnel: [w470] -> w439
          shift-right: [w467] -> _
          shift-left: _ -> [w468]
          tunnel: w437 -> [w467]
          tunnel: [w466] -> w436
          tunnel: w432 -> [w465]
          stop <- FALSE continue-if-true
          n213 = Not Equal?(x=w468, y=w467) -> (x != y?=w466:bool)
        }
        n214 = Not Equal?(x=w439, y=w440) -> (x != y?=w438:bool)
        n215 = And(x=w437, y=w436) -> (x .and. y?=w435:bool)
        n216 = Compound Arithmetic op=OR(w435, w438) -> (w419:bool)
        n217 = case shown="True" w419 {
          tunnel: [w442 "Plot3"] -> w420
          tunnel: w418 -> [w442 _]
          frame False {
          }
          frame True {
            n218 = property on="Plot 3 status" class="Str"("Visible"=TRUE) -> ()  [unwired: 2 in, 2 out]
          }
        }
        n219 = local read "Max Time"() -> (w423:timestamp)
        n220 = local read "Min Time"() -> (w424:timestamp)
        n221 = call "Selection_with_Search.vi"("Selected Channel Names"=w432, "Search String"="Search 3", "All Channel Names"=w433) -> ("Item Names"=w429:string[])
        n222 = for {
          tunnel: w429 -> [w453]
          tunnel: w432 -> [w452] mode=indexing
          tunnel: [w451] -> w430 mode=indexing
          n223 = Search 1D Array(1D array=w453, element=w452) -> (index of element=w451:i32)  [unwired: 1 out]
        }
        n224 = Not Equal?(x=w429, y=w425) -> (x != y?=w431:bool)
        n225 = To Double Precision Float(number=w423) -> (double precision float=w422:dbl)
        n226 = To Double Precision Float(number=w424) -> (double precision float=w421:dbl)
        n227 = case shown="True" w431 {
          tunnel: w430 -> [_ w450]
          tunnel: w429 -> [_ w449]
          frame False {
          }
          frame True {
            n228 = local write "Selector 3"(w450) -> ()
            n229 = property on="Selector 3" class="LstBox (strict)"("Item Names"=w449, "Top Row"=0) -> ()  [unwired: 2 in, 2 out]
          }
        }
        n230 = property on="Plot 3" class="XYGraph (strict)"("X Scale.Range:Maximum"=w422, "X Scale.Range:Minimum"=w421) -> ()  [unwired: 2 in, 2 out]
      }
      frame "Save Plot" {
        n231 = stacked-sequence {
          seq-local: [w489 _] -> [_ w525]
          seq-local: [w477 _] -> [_ w527]
          seq-local: [w475 _] -> [_ w526]
          tunnel: ["What to do next?" _] -> w472
          frame #0 {
            n232 = case shown="\"Save Plot 3\"" "Save plot number" {
              tunnel: [w502 w505 w508] -> w494
              tunnel: [w501 w504 w507] -> w489
              frame "Save Plot 1" {
                n233 = local read "Plot 1 Chs"() -> (w501:string[])
                n234 = local write "Save 1"(FALSE ("Save 1")) -> ()
                n235 = local read "Plot 1"() -> (w502:cluster{dbl[], "Output array":dbl[]}[])
              }
              frame "Save Plot 2" {
                n236 = local read "Plot 2 Chs"() -> (w504:string[])
                n237 = local write "Save 2"(FALSE ("Save 1")) -> ()
                n238 = local read "Plot 2"() -> (w505:cluster{"Times":dbl[], "Output array":dbl[]}[])
              }
              frame "Save Plot 3" {
                n239 = local read "Plot 3 Chs"() -> (w507:string[])
                n240 = local write "Save 3"(FALSE ("Save 1")) -> ()
                n241 = local read "Plot 3"() -> (w508:cluster{"Times":dbl[], "Output array":dbl[]}[])
              }
            }
            n242 = local read "Min Time"() -> (w488:timestamp)
            n243 = local read "Max Time"() -> (w486:timestamp)
            n244 = Index Array(array=w494, index=0) -> (element=w492:cluster{"Times":dbl[], "Output array":dbl[]})
            n245 = To Double Precision Float(number=w488) -> (double precision float=w484:dbl)
            n246 = To Double Precision Float(number=w486) -> (double precision float=w485:dbl)
            n247 = Unbundle(w492) -> ("Times"=w478:dbl[])  [unwired: 1 out]
            n248 = Threshold 1D Array(2:w484, 3:w478) -> (0:w487:dbl)  [unwired: 1 out]
            n249 = Threshold 1D Array(2:w485, 3:w478) -> (0:w483:dbl)  [unwired: 1 out]
            n250 = Round Toward -Infinity(1:w487) -> (0:w481:dbl)
            n251 = Round Toward +Infinity(x=w483) -> (ceil(x): smallest int >= x=w482:dbl)
            n252 = To Long Integer(number=w481) -> (32bit integer=w480:i32)
            n253 = Subtract(x=w482, y=w481) -> (x-y=w479:dbl)
            n254 = for {
              N: w479 -> [_]
              tunnel: w480 -> [w499]
              tunnel: w478 -> [w497]
              tunnel: [w496] -> w477 mode=indexing
              tunnel: [w495] -> w476 mode=indexing
              i -> [w498]
              n255 = Add(x=w499, y=w498) -> (x+y=w495:i32)
              n256 = Index Array(array=w497, index=w495) -> (element=w496:dbl)
            }
            n257 = for {
              tunnel: w494 -> [w512] mode=indexing
              tunnel: w476 -> [w511]
              tunnel: [w509] -> w475 mode=indexing
              n258 = Unbundle(w512) -> ("Output array"=w510:dbl[])  [unwired: 1 out]
              n259 = for {
                tunnel: w511 -> [w515] mode=indexing
                tunnel: w510 -> [w514]
                tunnel: [w513] -> w509 mode=indexing
                n260 = Index Array(array=w514, index=w515) -> (element=w513:dbl)
              }
            }
          }
          frame #1 {
            w520 = FALSE  # append to file? (new file:F)
            (unwired) T3."new file" ("select mode (2)")
            n261 = for {
              tunnel: w526 -> [w544]
              tunnel: w527 -> [w538] mode=indexing
              tunnel: [w540] -> w519 mode=indexing
              i -> [w543]
              n262 = Number To Decimal String(number=w538) -> (decimal integer string=w539:string)  [unwired: 1 out]
              n263 = Index Array(array=w544, index (col)=w543) -> (element=w542:dbl[])  [unwired: 1 in]
              n264 = Get Date/Time String(seconds (now)=w538) -> (date string=w537:string, time string=w536:string)  [unwired: 2 out]
              n265 = for {
                tunnel: w542 -> [w546] mode=indexing
                tunnel: [w545] -> w541 mode=indexing
                n266 = call "Number_2_string.vi"("number"=w546) -> ("String"=w545:string)  [unwired: 1 in]
              }
              n267 = Build Array (concatenate)(w537, w536, w539, w541) -> (w540:string[])
            }
            n268 = Build Array (concatenate)("Date::", "Centre:Time:", "Seconds:Since:1st Jan 1904", w525) -> (w518:string[])
            n269 = call "Ch_names_to_rows.vi"("Channel Names"=w518) -> ("3 Row names"=w524:string[][])
            n270 = File Dialog(7:"Please choose file name" ("prompt")) -> (3:w532:path)  [unwired: 1 in, 8 out]
            n271 = Build Array (concatenate)(w524, w519) -> (w522:string[][])
            n272 = Strip Path(path=w532) -> (stripped path=w529:path, name=w531:string)
            n273 = call "Add_filename_suffix.vi"("Filename"=w531, "Suffix to add"=".xls") -> ("Filename out"=w528:string)  [unwired: 3 out]
            n274 = Array To Spreadsheet String(array=w522, 3:"%s" ("format string")) -> (spreadsheet string=w521:string)  [unwired: 1 out]
            n275 = Build Path(base path=w529, name or relative path=w528) -> (appended path=w517:path)
            n276 = call "Write_File_Simple.vi"("append to file? (new file:F)"=w520, "character string"=w521, "file path"=w517) -> ()  [unwired: 2 out]
          }
        }
      }
      frame "What to do next?" {
        n277 = while {
          shift-right: [w584] -> _
          shift-left: _ -> [w583]
          shift-right: [w580] -> _
          shift-left: _ -> [w581]
          tunnel: w559 -> [w580]
          shift-right: [w578] -> _
          shift-left: _ -> [w579]
          tunnel: w561 -> [w578]
          tunnel: [w576] -> w560
          shift-right: [w574] -> w551
          shift-left: _ -> [w575]
          stop <- FALSE continue-if-true
          n278 = local read "History (days)"() -> (w584:i32)
          n279 = Not Equal?(x=w584, y=w583) -> (x != y?=w573:bool)
          n280 = Not Equal?(x=w580, y=w581) -> (x != y?=w577:bool)
          n281 = Not Equal?(x=w579, y=w578) -> (x != y?=w572:bool)
          n282 = Compound Arithmetic op=OR(w573, w577, w572, "Reload") -> (w576:bool)
          n283 = case shown="False" w576 {
            tunnel: w575 -> [w585 w588]
            tunnel: [w586 w588] -> w574
            frame False {
              n284 = Wait (ms)(milliseconds to wait=u32 100) -> ()  [unwired: 1 out]
              n285 = Increment(x=w585) -> (x+1=w586:dbl)
            }
            frame True {
            }
          }
          n286 = Compound Arithmetic op=OR(w573, w572, "Reload") -> (→"Change Scale?":bool)
        }
        n287 = Get Date/Time String(date format (0)=enum16{"short", "long", "abbreviated"}."abbreviated") -> (date string=w564:string, time string=w565:string)  [unwired: 2 out]
        n288 = Concatenate Strings(w564, " at " ("Substring"), w565) -> (→"Last Updated":string)
        n289 = Array Size(array=w557) -> (size(s)=w558:i32)
        n290 = Greater Than 0?(x=w558) -> (x > 0?=w556:bool)
        n291 = Select(t="Check for Zoom", s=w556, f="Get Channel Names") -> (s? t:f=w553:string)
        n292 = Quotient & Remainder(x=w551, y=500) -> (x-y*floor(x/y)=w550:i32)  [unwired: 1 out]
        n293 = Equal To 0?(x=w550) -> (x = 0?=w548:bool)
        n294 = Or(x=w548, y="stop") -> (x .or. y?=w547:bool)
        n295 = Select(t="Save Channel Names", s=w547, f=w553) -> (s? t:f=w568:string)
      }
      frame "Rescale plots?" {
        n296 = local read "Show Full Time?"() -> (w592:bool)
        n297 = local read "Change Scale?"() -> (w594:bool)
        n298 = Or(x=w594, y=w592) -> (x .or. y?=w593:bool)
        n299 = case shown="False" w593 {
          tunnel: ["What to do next?" "Update Plot1?"] -> w591
          tunnel: [w597 FALSE] -> w590
          tunnel: w589 -> [w597 _]
          frame False {
          }
          frame True {
            w600 = FALSE ("Show Full Time?")
            n300 = local write "Show Full Time?"(w600) -> ()
            n301 = local write "Change Scale?"(w600) -> ()
            n302 = local read "Max Memory"() -> (w602:timestamp)
            n303 = local read "Min Memory"() -> (w603:timestamp)
            n304 = local write "Max Time"(w602) -> ()
            n305 = local write "Min Time"(w603) -> ()
          }
        }
      }
      frame "Save Channel Names" {
        w604 = 10 ("y")
        n306 = Less?(x=w605, y=w604) -> (x < y?=w606:bool)
        n307 = stacked-sequence {
          seq-local: [w616 _ _] -> [_ w658 _]
          seq-local: [_ w655 _] -> [_ _ w669]
          tunnel: w614 -> [_ _ w670]
          tunnel: w613 -> [_ _ w666]
          tunnel: w610 -> [_ w654 _]
          tunnel: w606 -> [_ w642 _]
          tunnel: w605 -> [_ w641 _]
          tunnel: w604 -> [_ w640 _]
          frame #0 {
            n308 = for {
              N: 3 -> [_]
              shift-right: [w620] -> w616
              shift-left: string[][] [] -> [w622]
              i -> [w627]
              n309 = Increment(x=w627) -> (x+1=w624:i32)
              n310 = case shown="2" w624 {
                tunnel: [w634 w635 w637] -> w626
                tunnel: [w633 w636 w638] -> w618
                frame 1, Default {
                  n311 = local read "Selector 1"() -> (w634:i32[])
                  n312 = property on="Selector 1" class="LstBox (strict)"() -> ("Item Names"=w633:string[])  [unwired: 2 in, 2 out]
                }
                frame 2 {
                  n313 = property on="Selector 2" class="LstBox (strict)"() -> ("Item Names"=w636:string[])  [unwired: 2 in, 2 out]
                  n314 = local read "Selector 2"() -> (w635:i32[])
                }
                frame 3 {
                  n315 = local read "Selector 3"() -> (w637:i32[])
                  n316 = property on="Selector 3" class="LstBox (strict)"() -> ("Item Names"=w638:string[])  [unwired: 2 in, 2 out]
                }
              }
              n317 = Format Into String(format string="%d" ("Format String"), initial string="Selector ", w624) -> (resulting string=w621:string)  [unwired: 1 in, 1 out]
              n318 = for {
                tunnel: w626 -> [w632] mode=indexing
                tunnel: w621 -> [w631]
                tunnel: [w629] -> w619 mode=indexing
                tunnel: w618 -> [w628]
                n319 = Index Array(array=w628, index=w632) -> (element=w630:string)
                n320 = Build Array(w631, w630) -> (w629:string[])
              }
              n321 = Build Array (concatenate)(w622, w619) -> (w620:string[][])
            }
          }
          frame #1 {
            n322 = Select(t=w641, s=w642, f=w640) -> (s? t:f=w639:i32)
            n323 = local read "Data folder location"() -> (w645:path)
            n324 = local read "Search 1"() -> (w664:string)
            n325 = Number To Decimal String(number=w654) -> (decimal integer string=w652:string)  [unwired: 1 out]
            n326 = local read "Search 2"() -> (w661:string)
            n327 = Number To Decimal String(number=w639) -> (decimal integer string=w649:string)  [unwired: 1 out]
            n328 = local read "Search 3"() -> (w660:string)
            n329 = Path To String(path=w645) -> (string=w644:string)
            n330 = Build Array("Averaging Time (min)" ("element"), w652) -> (w650:string[])
            n331 = Build Array("Search 1 string" ("element"), w664) -> (w651:string[])
            n332 = Build Array("History in Days" ("element"), w649) -> (w647:string[])
            n333 = Build Array("Search 2 string" ("element"), w661) -> (w657:string[])
            n334 = Build Array("Search 3 string" ("element"), w660) -> (w656:string[])
            n335 = Build Array("Data folder location", w644) -> (w643:string[])
            n336 = Build Array (concatenate)(w658, w643, w647, w650, w651, w657, w656) -> (w655:string[][])
          }
          frame #2 {
            n337 = call "Setup_Filepath.vi"("Setup File Type"=Setup_Filetype."General", "Filename in"=w666) -> ("Filename Out"=w665:path)  [unwired: 1 out]
            n338 = Array Size(array=w669) -> (size(s)=w672:i32[])
            n339 = Index Array(array=w672, index=1 ("Index")) -> (element=w671:i32)
            n340 = Not Equal To 0?(x=w671) -> (x != 0?=w668:bool)
            n341 = case shown="True" w668 {
              tunnel: w665 -> [w674 w679]
              tunnel: w669 -> [_ w680]
              tunnel: w670 -> [_ w681]
              frame False {
                n342 = Delete(path (use dialog)=w674) -> ()  [unwired: 1 in, 6 out]
              }
              frame True {
                w675 = FALSE  # append to file? (new file:F)
                n343 = call "Ch_names_to_rows.vi"("Channel Names"=w681) -> ("3 Row names"=w682:string[][])
                n344 = Build Array (concatenate)(w682, w680) -> (w677:string[][])
                n345 = Array To Spreadsheet String(array=w677, 3:"%s" ("format string")) -> (spreadsheet string=w676:string)  [unwired: 1 out]
                n346 = call "Write_File_Simple.vi"("append to file? (new file:F)"=w675, "character string"=w676, "file path"=w679) -> ()  [unwired: 2 out]
              }
            }
          }
        }
        n347 = local read "stop"() -> (w608:bool)
        n348 = Not(x=w608) -> (.not. x?=w607:bool)
      }
    }
  }
